vi "interp_1d_nearest.vi"(9 "xi":dbl[](array[numeric]), 10 "X":dbl[](array[numeric]), 11 "Y":dbl[](array[numeric])) -> (3 "yi":dbl[](array[numeric]))   [LabVIEW 2019]
uses:
  <vilib>/gmath/NI_Gmath.lvlib
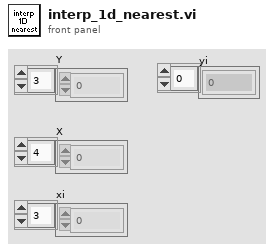
[diagram p1: front panel]
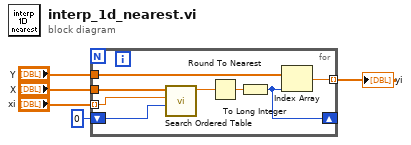
[diagram p0: block diagram]
diagram:
  n1 = for {
    tunnel: "X" -> [w10]
    tunnel: "xi" -> [w9] mode=indexing
    tunnel: "Y" -> [w12]
    tunnel: [w11] -> w3 mode=indexing
    shift-right: [w6] -> _
    shift-left: 0 -> [w8]
    n2 = call <vilib>:"Search Ordered Table.vi"("starting index"=w8, "x value"=w9, "ordered x array"=w10) -> ("fractional index"=w7:dbl)  [unwired: 8 in]
    n3 = Round To Nearest(number=w7) -> (nearest integer value=w13:dbl)
    n4 = To Long Integer(number=w13) -> (32bit integer=w6:i32)
    n5 = Index Array(array=w12, index=w6) -> (element=w11:dbl)
  }
  "yi" <- w3
